vi "sub2.vi"(10 "regular expression":string, 11 "Array":T1(array[cluster])) -> (3 "Tunnel out":refnum<vi>)   [LabVIEW 2020, in "CSM-Helper.lvclass"]
uses:
  CSM-Helper.lvclass
  CSM-Helper.lvclass/CSM-Helper.ctl
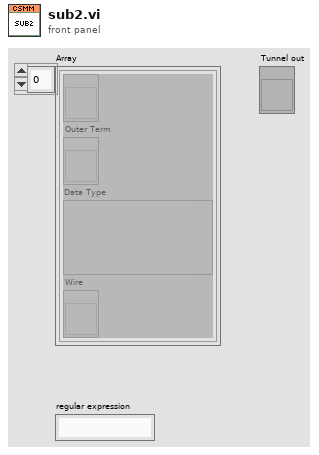
[diagram p1: front panel]
types:
  T1 = cluster{refnum<vi>, "Outer Term":refnum<vi>, "Data Type":variant, "Wire":refnum<vi>}[]
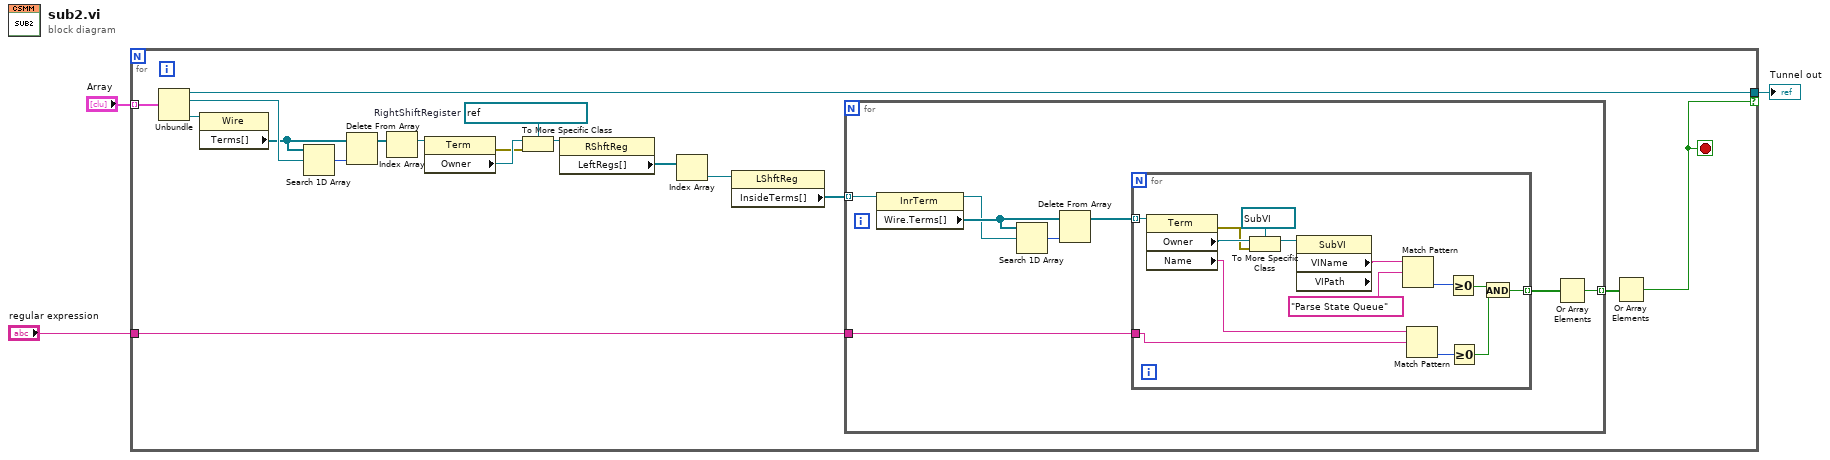
[diagram p0: block diagram]
diagram:
  n1 = for {
    tunnel: "Array" -> [w21] mode=indexing
    tunnel: [w20] -> w3 if=w11
    tunnel: "regular expression" -> [w10]
    stop <- w11 stop-if-true
    w17 = refnum<vi> refnum  # RightShiftRegister
    n2 = Unbundle(w21) -> (w20:refnum<vi>, "Outer Term"=w7:refnum<vi>, "Wire"=w19:refnum<vi>)  [unwired: 1 out]
    n3 = property class="Wire"(reference=w19) -> ("Terms[]"=w5:refnum<vi>[])  [unwired: 1 in, 2 out]
    n4 = Search 1D Array(1D array=w5, element=w7) -> (index of element=w6:i32)  [unwired: 1 in]
    n5 = Delete From Array(array=w5, index=w6) -> (array with subset deleted=w4:refnum<vi>[])  [unwired: 1 in, 1 out]
    n6 = Index Array(array=w4) -> (element=w18:refnum<vi>)  [unwired: 1 in]
    n7 = property class="Term"(reference=w18) -> (error out=w8:errorcluster, "Owner"=w9:refnum<vi>)  [unwired: 1 in, 1 out]
    n8 = To More Specific Class(target class=w17, reference=w9, error in=w8) -> (specific class reference=w16:refnum<vi>)  [unwired: 1 out]
    n9 = property class="RShftReg"(reference=w16) -> ("LeftRegs[]"=w15:refnum<vi>[])  [unwired: 1 in, 2 out]
    n10 = Index Array(array=w15) -> (element=w14:refnum<vi>)  [unwired: 1 in]
    n11 = property class="LShftReg"(reference=w14) -> ("InsideTerms[]"=w13:refnum<vi>[])  [unwired: 1 in, 2 out]
    n12 = for {
      tunnel: w13 -> [w29] mode=indexing
      tunnel: [w27] -> w12 mode=indexing
      tunnel: w10 -> [w26]
      n13 = property class="InrTerm"(reference=w29) -> (reference out=w22:refnum<vi>, "Wire.Terms[]"=w24:refnum<vi>[])  [unwired: 1 in, 1 out]
      n14 = Search 1D Array(1D array=w24, element=w22) -> (index of element=w25:i32)  [unwired: 1 in]
      n15 = Delete From Array(array=w24, index=w25) -> (array with subset deleted=w23:refnum<vi>[])  [unwired: 1 in, 1 out]
      n16 = for {
        tunnel: [w32] -> w28 mode=indexing
        tunnel: w23 -> [w31] mode=indexing
        tunnel: w26 -> [w30]
        n17 = property class="Term"(reference=w31) -> (error out=w41:errorcluster, "Owner"=w43:refnum<vi>, "Name"=w37:string)  [unwired: 1 in, 1 out]
        n18 = To More Specific Class(target class=refnum<vi> refnum ("Parse State Queue"), reference=w43, error in=w41) -> (specific class reference=w40:refnum<vi>)  [unwired: 1 out]
        n19 = property class="SubVI" props=["VIName", "VIPath"](reference=w40) -> ("VIName"=w39:string)  [unwired: 1 in, 3 out]
        n20 = Match Pattern(string=w39, regular expression="Parse State Queue") -> (offset past match=w36:i32)  [unwired: 1 in, 3 out]
        n21 = Match Pattern(string=w37, regular expression=w30) -> (offset past match=w35:i32)  [unwired: 1 in, 3 out]
        n22 = Greater Or Equal To 0?(x=w36) -> (x >= 0?=w34:bool)
        n23 = Greater Or Equal To 0?(x=w35) -> (x >= 0?=w33:bool)
        n24 = And(x=w34, y=w33) -> (x .and. y?=w32:bool)
      }
      n25 = Or Array Elements(Boolean array=w28) -> (logical OR=w27:bool)
    }
    n26 = Or Array Elements(Boolean array=w12) -> (logical OR=w11:bool)
  }
  "Tunnel out" <- w3
